vi "briefcase.vi"() -> ()   [LabVIEW 2011]
uses:
  <vilib>/Utility/config.llb/Read Key (String).vi
  <vilib>/Utility/config.llb/Read Key (I32).vi
  <vilib>/Utility/inputDevices.llb/closeKeyboard.vi
  <vilib>/Utility/config.llb/NI_LVConfig.lvlib
panel:
  out "Good connection":bool
  out "Host ping":bool
  out "Current":T1
  in  "Disable":T1
  in  "Enable":T1
  in  "Disable":T2
  out "Current":T2
  in  "Enable":T2
  in  "stop":bool
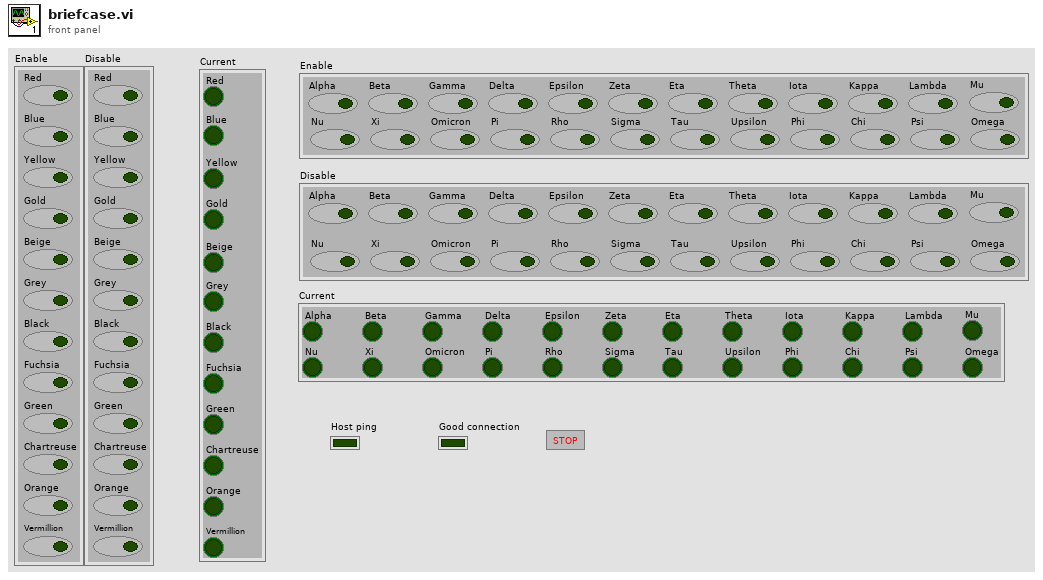
[diagram p1: front panel]
types:
  T1 = cluster{"Alpha":bool, "Beta":bool, "Gamma":bool, "Delta":bool, "Epsilon":bool, "Zeta":bool, "Eta":bool, "Theta":bool, "Iota":bool, "Kappa":bool, "Lambda":bool, "Mu":bool, "Nu":bool, "Xi":bool, "Omicron":bool, "Pi":bool, "Rho":bool, "Sigma":bool, "Tau":bool, "Upsilon":bool, "Phi":bool, "Chi":bool, "Psi":bool, "Omega":bool}
  T2 = cluster{"Red":bool, "Blue":bool, "Yellow":bool, "Gold":bool, "Beige":bool, "Grey":bool, "Black":bool, "Fuchsia":bool, "Green":bool, "Chartreuse":bool, "Orange":bool, "Vermillion":bool}
  T3 = typedef "NI_LVConfig.lvlib/Config Data RefNum.ctl" = refnum<k1>
  T4 = typedef "LVAllMonitorsDisplayTypeDef.ctl" = cluster{"Bounds":cluster{"Left":i16, "Top":i16, "Right":i16, "Bottom":i16}, "Depth":i16}[]
  T5 = cluster{"Bounds":cluster{"Left":i16, "Top":i16, "Right":i16, "Bottom":i16}, "Depth":i16}
  T6 = cluster{"Left":i16, "Top":i16, "Right":i16, "Bottom":i16}
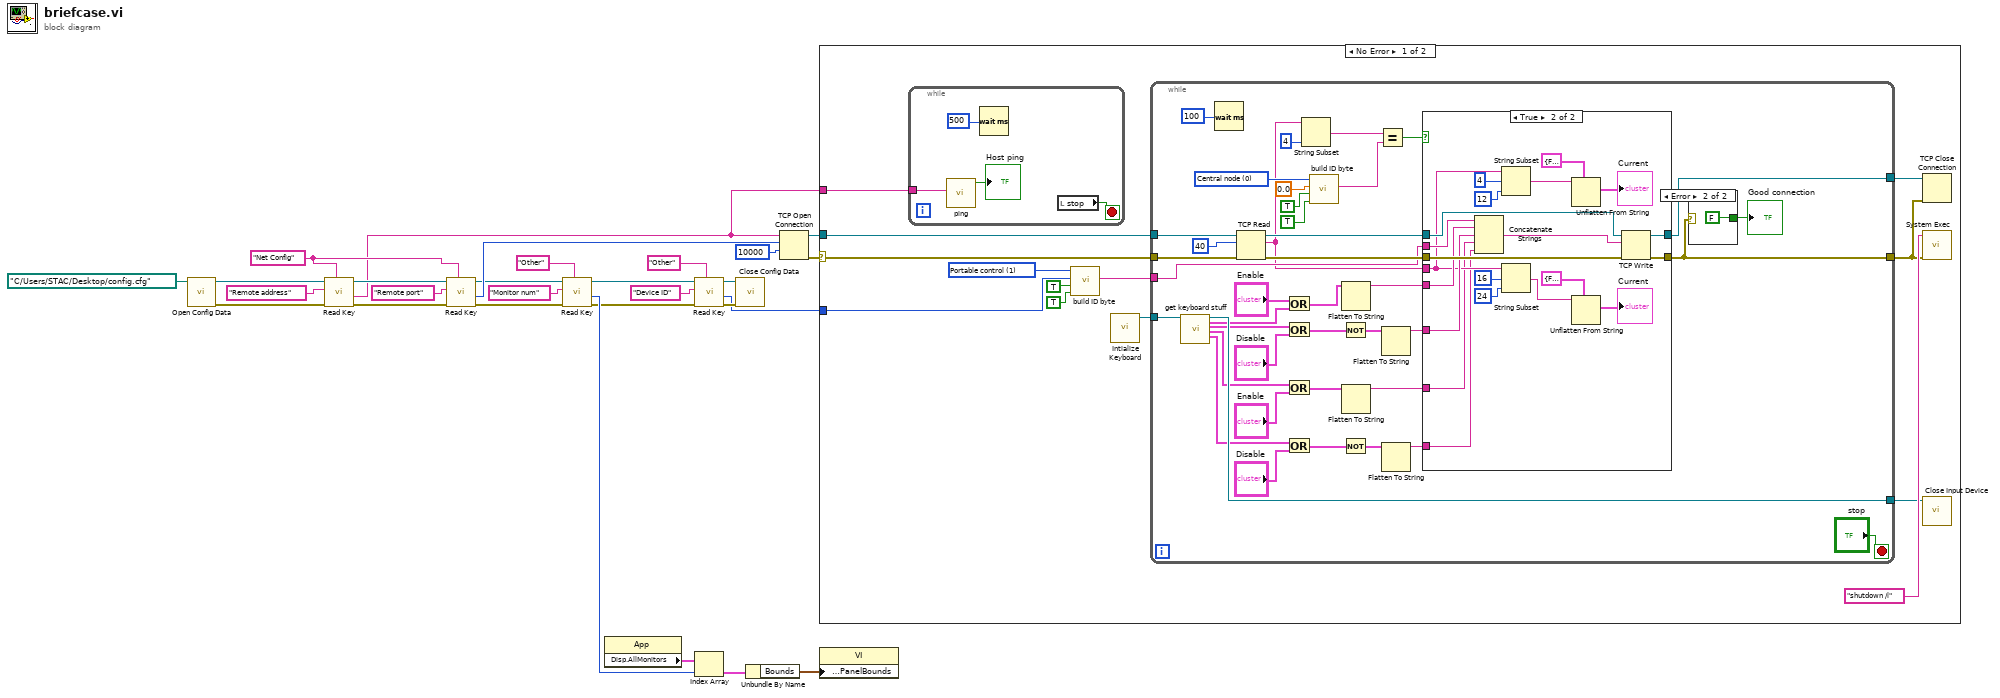
[diagram p0: block diagram]
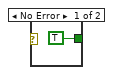
[diagram p3: hidden frame]
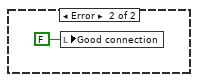
[diagram p4: hidden frame]
diagram:
  w18 = "Net Config" ("section")
  n1 = call <vilib>:"Open Config Data.vi"("configuration file path"=path "C:/Users/STAC/Desktop/config.cfg") -> ("error out"=w25:errorcluster, "refnum"=w26:T3)  [unwired: 8 in, 1 out]
  n2 = call-poly <vilib>:"Read Key.vi"("section"=w18, "error in (no error)"=w25, "key"="Remote address", "refnum"=w26) -> ("error out"=w21:errorcluster, "value"=w16:string, "refnum out"=w22:T3)  [unwired: 4 in, 1 out]
  n3 = call-poly <vilib>:"Read Key.vi"("section"=w18, "error in (no error)"=w21, "key"="Remote port", "refnum"=w22) -> ("error out"=w14:errorcluster, "value"=w19:i32, "refnum out"=w15:T3)  [unwired: 4 in, 1 out]
  n4 = call-poly <vilib>:"Read Key.vi"("section"="Other", "error in (no error)"=w14, "key"="Monitor num", "refnum"=w15) -> ("error out"=w5:errorcluster, "value"=w8:i32, "refnum out"=w6:T3)  [unwired: 4 in, 1 out]
  n5 = property class="App"() -> ("Disp.AllMonitors"=w11:T4)  [unwired: 2 in, 2 out]
  n6 = call-poly <vilib>:"Read Key.vi"("section"="Other", "error in (no error)"=w5, "key"="Device ID", "refnum"=w6) -> ("error out"=w4:errorcluster, "value"=w2:i32, "refnum out"=w7:T3)  [unwired: 4 in, 1 out]
  n7 = Index Array(array=w11, index=w8) -> (element=w10:T5)
  n8 = call <vilib>:"Close Config Data.vi"("error in (no error)"=w4, "refnum"=w7) -> ()  [unwired: 8 in, 2 out]
  n9 = Unbundle By Name(w10) -> ("Bounds"=w9:T6)
  n10 = TCP Open Connection(address=w16, remote port or service name=w19, timeout ms (60000)=10000) -> (connection ID=w28:refnum<k5>, error out=w17:errorcluster)  [unwired: 2 in]
  n11 = case shown="No Error" w17 {
    selector: w17 -> [w34 _]
    tunnel: w28 -> [w35 _]
    tunnel: w2 -> [w37 _]
    tunnel: w16 -> [w33 _]
    frame No Error {
      w38 = u16 1 items=["Central node", "Portable control", "Boolean sensor", "Boolean output", "8-bit sensor", "8-bit output"] ("Type")
      n12 = while {
        tunnel: w33 -> [w45]
        stop <- w42 stop-if-true
        n13 = call "ping.vi"("Remote address"=w45) -> ("Connection?"=→"Host ping":bool)  [unwired: 9 in, 1 out]
        n14 = Wait (ms)(milliseconds to wait=u32 500) -> ()  [unwired: 1 out]
        n15 = local read "stop"() -> (w42:bool)
      }
      n16 = call "build ID byte.vi"("Output?"=TRUE, "Input?"=TRUE, "Node ID"=w37, "Type"=w38) -> ("ID byte"=w36:string)  [unwired: 6 in, 1 out]
      n17 = call <vilib>:"Intialize Keyboard.vi"() -> ("device ID"=w30:refnum<k1>)  [unwired: 10 in, 1 out]
      n18 = while {
        tunnel: w35 -> [w85]
        tunnel: [w73] -> w41
        tunnel: w34 -> [w83]
        tunnel: [w72] -> w31
        tunnel: w36 -> [w69]
        tunnel: w30 -> [w58]
        tunnel: [w59] -> w29
        stop <- "stop" stop-if-true
        w81 = u16 0 items=["Central node", "Portable control", "Boolean sensor", "Boolean output", "8-bit sensor", "8-bit output"] ("Type")
        n19 = call "get keyboard stuff.vi"("Keyboard Ref In"=w58) -> ("Keyboard Ref Out"=w59:refnum<k1>, "Engage Codes"=w55:T2, "Disengage Codes"=w52:T2, "Engage Protocols"=w49:T1, "Disengage Protocols"=w46:T1)  [unwired: 14 in]
        n20 = Wait (ms)(milliseconds to wait=u32 100) -> ()  [unwired: 1 out]
        n21 = TCP Read(connection ID=w85, bytes to read=40, error in (no error)=w83) -> (connection ID out=w71:refnum<k5>, data out=w66:string, error out=w70:errorcluster)  [unwired: 2 in]
        n22 = Or(x="Enable", y=w55) -> (x .or. y?=w57:T2)
        n23 = Or(x=w52, y="Disable") -> (x .or. y?=w54:T2)
        n24 = Or(x=w49, y="Enable") -> (x .or. y?=w51:T1)
        n25 = Or(x=w46, y="Disable") -> (x .or. y?=w48:T1)
        n26 = String Subset(string=w66, length (rest)=4 ("length (rest)")) -> (substring=w76:string)  [unwired: 1 in]
        n27 = call "build ID byte.vi"("Output?"=TRUE, "Input?"=TRUE, "Node ID"=0.0, "Type"=w81) -> ("ID byte"=w75:string)  [unwired: 6 in, 1 out]
        n28 = Not(x=w54) -> (.not. x?=w60:T2)
        n29 = Not(x=w48) -> (.not. x?=w61:T1)
        n30 = Flatten To String(anything=w57) -> (data string=w68:string)  [unwired: 3 in, 2 out]
        n31 = Flatten To String(anything=w51) -> (data string=w65:string)  [unwired: 3 in, 2 out]
        n32 = Equal?(x=w76, y=w75) -> (x = y?=w74:bool)
        n33 = Flatten To String(anything=w60) -> (data string=w67:string)  [unwired: 3 in, 2 out]
        n34 = Flatten To String(anything=w61) -> (data string=w64:string)  [unwired: 3 in, 2 out]
        n35 = case shown="True" w74 {
          tunnel: [w87 w108] -> w73
          tunnel: [w86 w107] -> w72
          tunnel: w71 -> [w87 w106]
          tunnel: w70 -> [w86 w105]
          tunnel: w69 -> [_ w104]
          tunnel: w67 -> [_ w103]
          tunnel: w68 -> [_ w102]
          tunnel: w66 -> [_ w96]
          tunnel: w65 -> [_ w90]
          tunnel: w64 -> [_ w89]
          frame False {
          }
          frame True {
            n36 = Concatenate Strings(w104, w102, w103, w90, w89) -> (w88:string)
            n37 = String Subset(string=w96, offset (0)=4, length (rest)=12 ("length (rest)")) -> (substring=w100:string)
            n38 = String Subset(string=w96, offset (0)=16, length (rest)=24 ("length (rest)")) -> (substring=w93:string)
            n39 = Unflatten From String(type=T2 {"Red"=FALSE, "Blue"=FALSE, "Yellow"=FALSE, "Gold"=FALSE, "Beige"=FALSE, "Grey"=FALSE, "Black"=FALSE, "Fuchsia"=FALSE, "Green"=FALSE, "Chartreuse"=FALSE, "Orange"=FALSE, "Vermillion"=FALSE}, binary string=w100) -> (value=→"Current":T2)  [unwired: 3 in, 2 out]
            n40 = Unflatten From String(type=T1 {"Alpha"=FALSE, "Beta"=FALSE, "Gamma"=FALSE, "Delta"=FALSE, "Epsilon"=FALSE, "Zeta"=FALSE, "Eta"=FALSE, "Theta"=FALSE, "Iota"=FALSE, "Kappa"=FALSE, "Lambda"=FALSE, "Mu"=FALSE, "Nu"=FALSE, "Xi"=FALSE, "Omicron"=FALSE, "Pi"=FALSE, "Rho"=FALSE, "Sigma"=FALSE, "Tau"=FALSE, "Upsilon"=FALSE, "Phi"=FALSE, "Chi"=FALSE, "Psi"=FALSE, "Omega"=FALSE}, binary string=w93) -> (value=→"Current":T1)  [unwired: 3 in, 2 out]
            n41 = TCP Write(connection ID=w106, data in=w88, error in (no error)=w105) -> (connection ID out=w108:refnum<k5>, error out=w107:errorcluster)  [unwired: 1 in, 1 out]
          }
        }
        n42 = case shown="Error" w72 {
          tunnel: [TRUE FALSE] -> w84
          frame No Error {
          }
          frame Error {
          }
        }
        "Good connection" <- w84
      }
      n43 = TCP Close Connection(connection ID=w41, error in (no error)=w31) -> ()  [unwired: 1 in, 2 out]
      n44 = call <vilib>:"System Exec.vi"("error in (no error)"=w31, "command line"="shutdown /l") -> ()  [unwired: 6 in, 4 out]
      n45 = call-poly <vilib>:"Close Input Device.vi"("device ID"=w29) -> ()  [unwired: 9 in, 1 out]
    }
    frame Error {
      n46 = local write "Good connection"(FALSE ("Good connection")) -> ()
    }
  }
  n47 = property class="VI"("Front Panel.PanelBounds"=w9) -> ()  [unwired: 2 in, 2 out]
